vi "Perform Action.vi"(8 "error in":errorcluster, 10 "Input":variant, 11 "Virt Instrument Base in":refnum<class "Virt Red-y Read Write.lvclass">) -> (0 "error out":errorcluster, 2 "Output":variant, 3 "Virt Instrument Base out":refnum<class "Virt Red-y Read Write.lvclass">)   [LabVIEW 2023, in "Virt Red-y Read Write.lvclass"]
uses:
  Virt Red-y Read Write.lvclass
  D:/git/HAL/HAL GOOP4/Virt Instr Base/Virt Instr Base.lvclass
  D:/git/HAL/HAL GOOP4/Virt Instr Host/Virt Instr Local.lvclass
  Configurations/Read Write CFG/Read Write PE Input.ctl
  <userlib>/_OpenG.lib/lvdata/lvdata.llb/Type Descriptor Enumeration__ogtk.ctl
  Virt Instr Host/Virt Instr Local.lvclass/Virt Instr Local.ctl
  Virt Instr Base/Virt Instr Base.lvclass/Virt Instr Base.ctl
  476c21fd-da13-441f-872e-21236ed22386.vi
  <vilib>/JDP Science/JSONtext/JSON text to Variant.vi
  <vilib>/Utility/error.llb/Error Cluster From Error Code.vi
  <vilib>/JDP Science/JSONtext/LVClass Serializer/JSONtext LVClass Serializer.lvclass
  <vilib>/ErrorRing/Error Ring.xnode
  Virt Red-y Read Write.lvclass/Virt Red-y Read Write.ctl
  Instrument/Instrument.lvclass
  Virt Instr Base/Virt Instr Base.lvclass
  Virt Instr Host/Virt Instr Local.lvclass
  D:/git/HAL/HAL GOOP4/Red-y/Virtual Instrs/Virt Red-y Read Write/Virt Red-y Read Write.lvclass
  <userlib>/_OpenG.lib/lvdata/lvdata.llb/openg_variant.lvlib
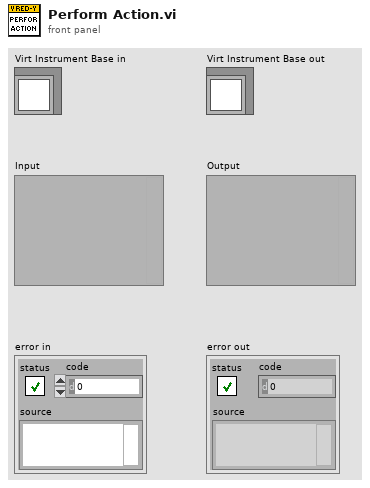
[diagram p1: front panel]
types:
  T1 = typedef "openg_variant.lvlib/Type Descriptor Enumeration__ogtk.ctl" = enum8{"<Null>", "I8", "I16", "I32", "I64", "U8", "U16", "U32", "U64", "SGL", "DBL", "EXT", "CSG", "CDB", "CXT", "0x0F", "0x10", "0x11", "0x12", "0x13", "0x14", "Enum U8", "Enum U16", "Enum U32", "Enum U64", "SGL PQ", "DBL PQ", "EXT PQ", "CSG PQ", "CDB PQ", "CXT PQ", "0x1F", "0x20", "Boolean", "0x22", "0x23", "0x24", "0x25", "0x26", "0x27", "0x28", "0x29", "0x2A", "0x2B", "0x2C", "0x2D", "0x2E", "0x2F", "String", "0x31", "Path", "Pict", "0x34", "0x35", "0x36", "DAQ", "0x38", "0x39", "0x3A", "0x3B", "0x3C", "0x3D", "0x3E", "0x3F", "Array", "0x41", "0x42", "0x43", "0x44", "0x45", "0x46", "0x47", "0x48", "0x49", "0x4A", "0x4B", "0x4C", "0x4D", "0x4E", "0x4F", "Cluster", "0x51", "0x52", "Variant", "Waveform", "0x55", "0x56", "0x57", "0x58", "0x59", "0x5A", "0x5B", "0x5C", "0x5D", "0x5E", "Fixed Point", "0x60", "0x61", "0x62", "0x63", "0x64", "0x65", "0x66", "0x67", "0x68", "0x69", "0x6A", "0x6B", "0x6C", "0x6D", "0x6E", "0x6F", "Refnum", "0x71", "0x72", "Set Collection", "Map Collection"}
  T2 = cluster{"Action":enum16{"Write", "Read"}, "Register":string, "Type":string}
  T3 = typedef "Read Write PE Input.ctl" = cluster{"Action":enum16{"Write", "Read"}, "Register":u16, "Type":T1, "Data":variant}
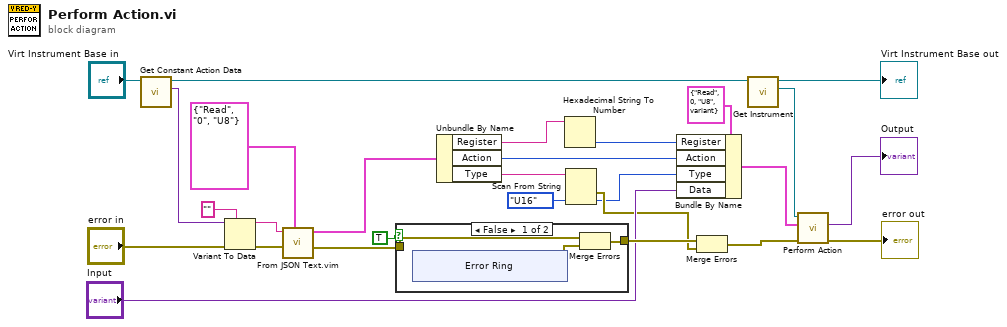
[diagram p0: block diagram]
diagram:
  n1 = call "Get Constant Action Data.vi"("Virt Instr Base in"="Virt Instrument Base in") -> ("Constant Action Data"=w19:variant, "Virt Instr Base out"=w24:refnum<class "Virt Red-y Read Write.lvclass">)  [unwired: 9 in]
  n2 = Variant To Data(error in="error in", type="", Variant=w19) -> (data=w7:string, error out=w8:errorcluster)
  n3 = call "From JSON Text.vim"("Data Type and Default Value"=T2 {"Action"=enum."Read", "Register"="0", "Type"="U8"}, "error in (no error)"=w8, "JSON"=w7) -> ("error out"=w17:errorcluster, "Data out"=w5:T2)  [unwired: 7 in]
  n4 = case shown="False" TRUE {
    tunnel: w17 -> [w29 w36]
    tunnel: [w30 w36] -> w16
    frame False {
      n5 = xnode "Error Ring"() -> ("error out"=w28:errorcluster)
      n6 = Merge Errors(w29, w28) -> (w30:errorcluster)
    }
    frame True {
    }
  }
  n7 = Unbundle By Name(w5) -> ("Register"=w2:string, "Action"=w3:enum16{"Write", "Read"}, "Type"=w13:string)
  n8 = Hexadecimal String To Number(string=w2) -> (number=w1:u32)  [unwired: 2 in, 1 out]
  n9 = Scan From String(input string=w13, default 1=Type_Descriptor_Enumeration__ogtk."U16" ("Type")) -> (error out=w10:errorcluster, output 1=w9:T1)  [unwired: 3 in, 2 out]
  n10 = Bundle By Name(cluster=T3 {"Action"=enum."Read", "Register"=0, "Type"=enum."U8", "Data"=variant} ("Cluster"), "Register"=w1, "Action"=w3, "Type"=w9, "Data"="Input") -> (w15:T3)
  n11 = Merge Errors(w16, w10) -> (w11:errorcluster)
  n12 = call "Get Instrument.vi"("Virt Instr Base in"=w24) -> ("HAL GOOP4.lvlib:Instrument"=w23:refnum<class "Instrument.lvclass">, "Virt Instr Base out"=→"Virt Instrument Base out":refnum<class "Virt Red-y Read Write.lvclass">)  [unwired: 9 in]
  n13 = call "Perform Action.vi"("Error In"=w11, "Input"=w15, "reference in"=w23) -> ("Error Out"=→"error out":errorcluster, "Output"=→"Output":variant)  [unwired: 6 in, 1 out]
